vi "Human Readable Error Message.vi"(3 "error in (no error)":errorcluster) -> (5 "Human readable error message":string)   [LabVIEW 2021, in "CIFCoreCommon.lvlib"]
uses:
  CIFCoreCommon.lvlib
  <vilib>/Utility/error.llb/whitespace.ctl
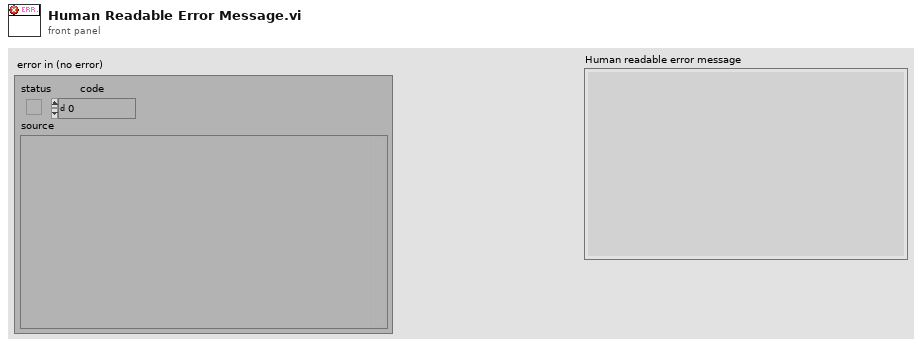
[diagram p1: front panel]
types:
  T1 = typedef "TagReturnType.ctl" = enum16{"No Tag", "<err>", "<append>"}
  T2 = typedef "whitespace.ctl" = u16
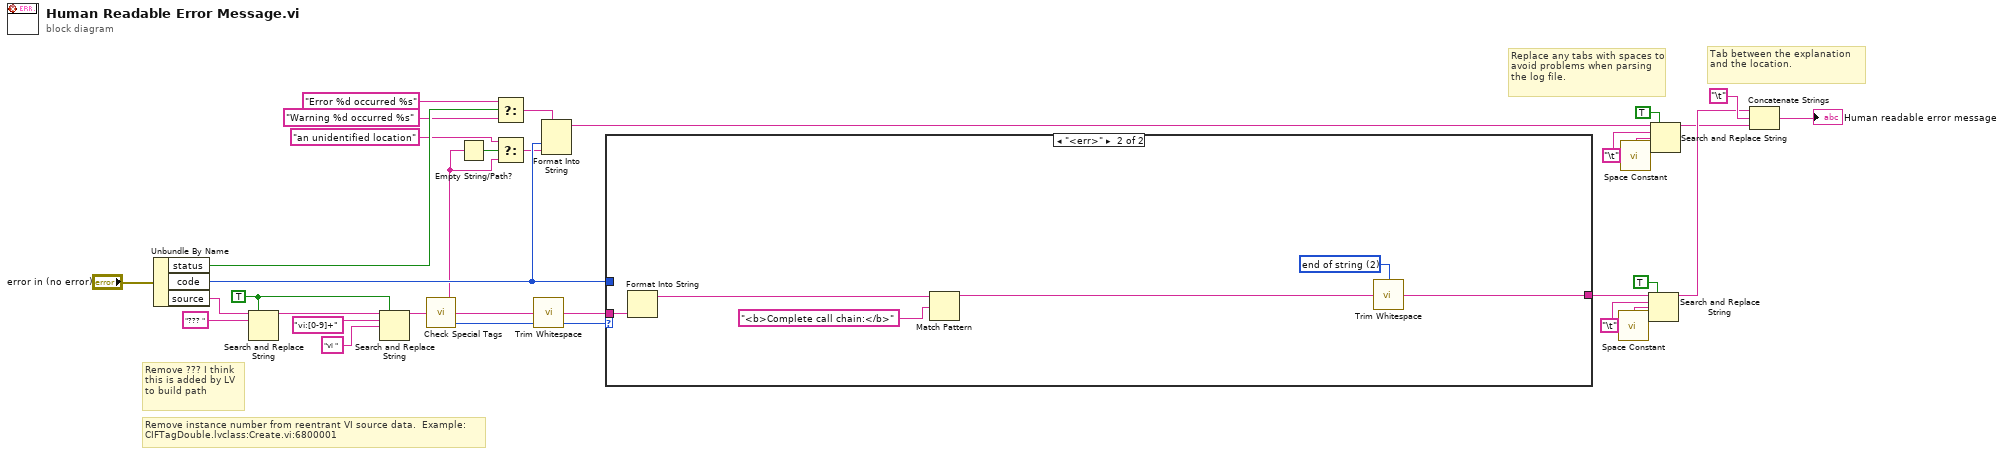
[diagram p0: block diagram]
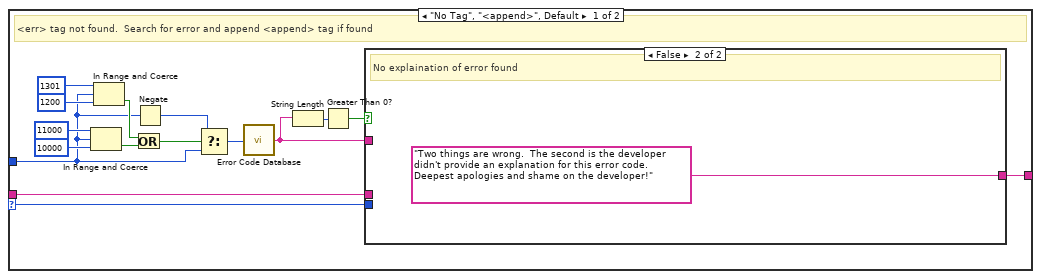
[diagram p2: hidden frame]
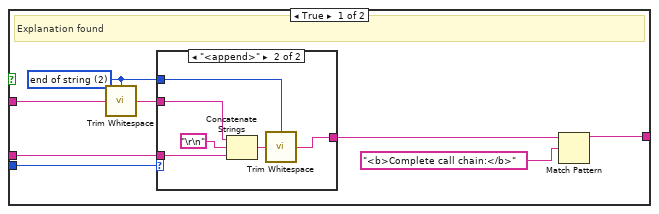
[diagram p3: hidden frame]
diagram:
  w15 = TRUE ("replace all? (F)")
  # "Tab between the explanation and the location."
  # "Replace any tabs with spaces to avoid problems when parsing the log file."
  # "Remove instance number from reentrant VI source data.  Example: \nCIFTagDouble.lvclass:Create.vi:6800001"
  # "Remove ??? I think this is added by LV to build path"
  n1 = Unbundle By Name("error in (no error)") -> ("status"=w25:bool, "code"=w32:i32, "source"=w21:string)
  n2 = Search and Replace String(replace all?=w15, input string=w21, search string="??? ") -> (result string=w17:string)  [unwired: 5 in, 3 out]
  n3 = Search and Replace String(replace all?=w15, input string=w17, search string="vi:[0-9]+" ("regular expression"), replace string="vi " ("replace string (\"\")")) -> (result string=w16:string)  [unwired: 4 in, 3 out]
  n4 = call <vilib>:"Check Special Tags.vi"("source"=w16) -> ("Before Tag (source)"=w27:string, "After Tag (special data)"=w2:string, "Tag Found?"=w26:T1)
  n5 = Empty String/Path?(string/path=w27) -> (empty?=w30:bool)
  n6 = Select(t="Error %d occurred %s" ("Error %d occurred at %s"), s=w25, f="Warning %d occurred %s" ("Warning %d occurred at %s")) -> (s? t:f=w29:string)
  n7 = Select(t="an unidentified location" ("an unidentified location"), s=w30, f=w27) -> (s? t:f=w28:string)
  n8 = call <vilib>:"Trim Whitespace.vi"("string"=w2) -> ("trimmed string"=w1:string)  [unwired: 1 in]
  n9 = Format Into String(format string=w29, w32, w28) -> (resulting string=w5:string)  [unwired: 2 in, 1 out]
  n10 = case shown="\"<err>\"" w26 {
    selector: w26 -> [w36 _]
    tunnel: w32 -> [w37 _]
    tunnel: w1 -> [w39 w70]
    tunnel: [w33 w68] -> w10
    frame "No Tag", "<append>", Default {
      # "<err> tag not found.  Search for error and append <append> tag if found"
      n11 = In Range and Coerce(upper limit=11000, x=w37, lower limit=10000) -> (In Range?=w43:bool)  [unwired: 1 out]
      n12 = In Range and Coerce(upper limit=1301, x=w37, lower limit=1200) -> (In Range?=w44:bool)  [unwired: 1 out]
      n13 = Or(x=w44, y=w43) -> (x .or. y?=w42:bool)
      n14 = Negate(x=w37) -> (-x=w46:i32)
      n15 = Select(t=w46, s=w42, f=w37) -> (s? t:f=w38:i32)
      n16 = call <vilib>:"Error Code Database.vi"("Error Code"=w38) -> ("Error Text"=w34:string)
      n17 = String Length(string=w34) -> (length=w40:i32)
      n18 = Greater Than 0?(x=w40) -> (x > 0?=w35:bool)
      n19 = case shown="False" w35 {
        tunnel: w34 -> [w53 _]
        tunnel: w36 -> [w54 _]
        tunnel: w39 -> [w55 _]
        tunnel: [w50 "Two things are wrong.  The second is the developer didn't provide an explanation for this error code. Deepest apologies and shame on the developer!" ("Error not listed")] -> w33
        frame True {
          w52 = T2 2 items=["both", "start of string", "end of string"] ("location (both)")
          # "Explanation found"
          n20 = call <vilib>:"Trim Whitespace.vi"("string"=w53, "location (both)"=w52) -> ("trimmed string"=w56:string)
          n21 = case shown="\"<append>\"" w54 {
            tunnel: w56 -> [w57 w63]
            tunnel: [w57 w61] -> w51
            tunnel: w55 -> [_ w60]
            tunnel: w52 -> [_ w58]
            frame "No Tag", Default {
            }
            frame "<append>" {
              n22 = Concatenate Strings(w63, "\r\n" ("End of Line Constant"), w60) -> (w62:string)
              n23 = call <vilib>:"Trim Whitespace.vi"("string"=w62, "location (both)"=w58) -> ("trimmed string"=w61:string)
            }
          }
          n24 = Match Pattern(string=w51, regular expression="<b>Complete call chain:</b>") -> (before substring=w50:string)  [unwired: 1 in, 3 out]
        }
        frame False {
          # "No explaination of error found"
        }
      }
    }
    frame "<err>" {
      w69 = T2 2 items=["both", "start of string", "end of string"] ("location (both)")
      n25 = Format Into String(w70) -> (resulting string=w66:string)  [unwired: 3 in, 1 out]
      n26 = Match Pattern(string=w66, regular expression="<b>Complete call chain:</b>") -> (before substring=w65:string)  [unwired: 1 in, 3 out]
      n27 = call <vilib>:"Trim Whitespace.vi"("string"=w65, "location (both)"=w69) -> ("trimmed string"=w68:string)
    }
  }
  n28 = call <vilib>:"Space Constant.vi"() -> ("String"=w11:string)
  n29 = call <vilib>:"Space Constant.vi"() -> ("String"=w7:string)
  n30 = Search and Replace String(replace all?=TRUE ("replace all? (F)"), input string=w10, search string="\t", replace string=w11) -> (result string=w9:string)  [unwired: 4 in, 3 out]
  n31 = Search and Replace String(replace all?=TRUE ("replace all? (F)"), input string=w5, search string="\t", replace string=w7) -> (result string=w4:string)  [unwired: 4 in, 3 out]
  n32 = Concatenate Strings(w9, "\t", w4) -> (→"Human readable error message":string)
